vi "Test Comparison.vi"(8 "error in":errorcluster) -> (0 "error out":errorcluster)   [LabVIEW 2013]
uses:
  <vilib>/addons/_JKI Toolkits/Caraya/classes/Test/Test.lvclass
  <vilib>/addons/_JKI Toolkits/Caraya/classes/Assert/Assert.lvclass
  <vilib>/addons/_JKI Toolkits/Caraya/classes/Assert/Assert True.vi
  source/Timestamp Compare Units -- enum.ctl
  <vilib>/addons/_JKI Toolkits/Caraya/classes/Assert/Assert False.vi
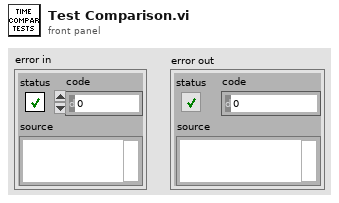
[diagram p1: front panel]
types:
  T1 = typedef "Timestamp Compare Units -- enum.ctl" = enum16{"week", "day", "hour", "minute", "second", "millisecond", "microsecond", "nanosecond"}
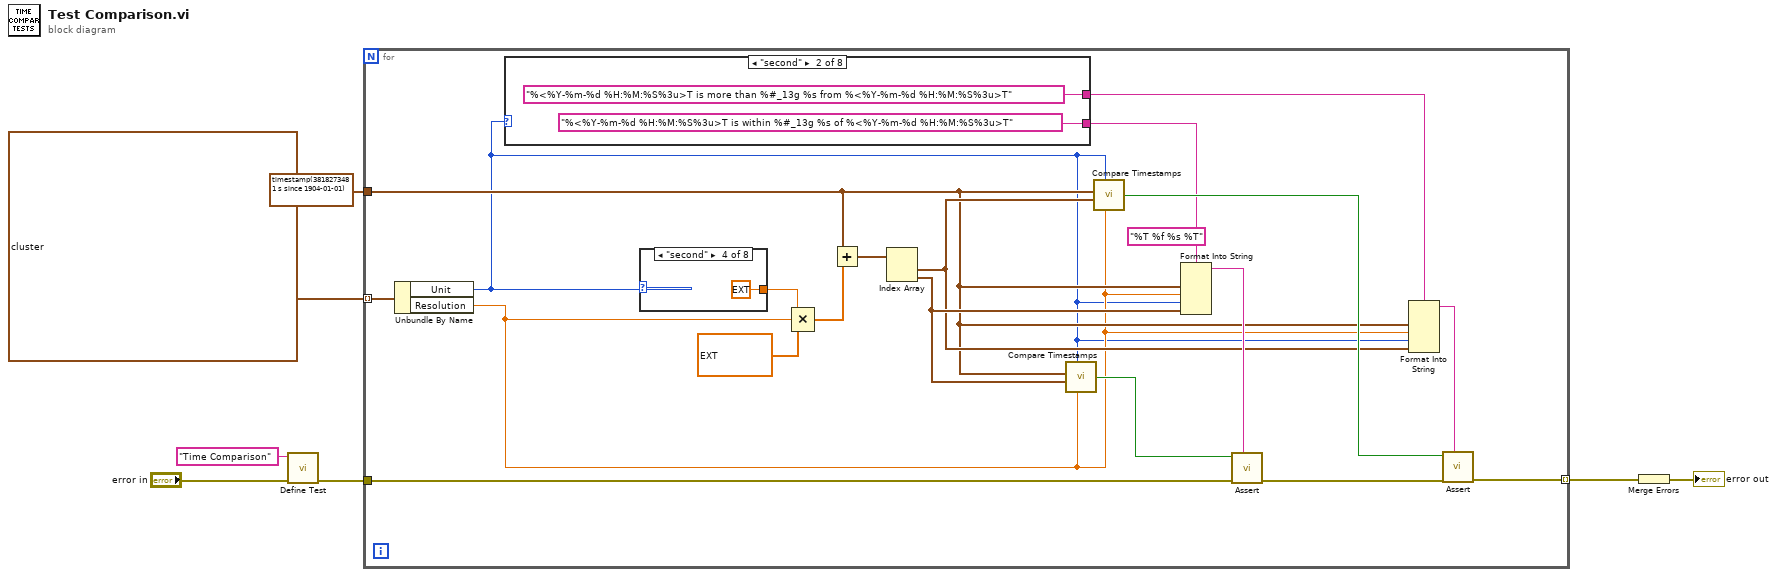
[diagram p0: block diagram]
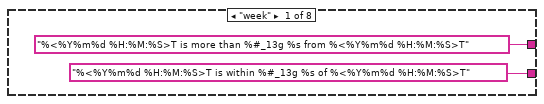
[diagram p2: hidden frame]
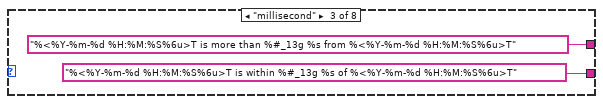
[diagram p3: hidden frame]
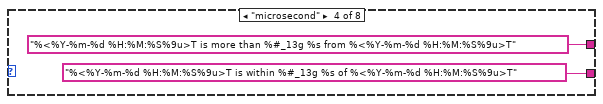
[diagram p4: hidden frame]
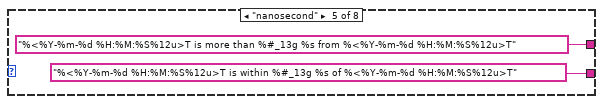
[diagram p5: hidden frame]
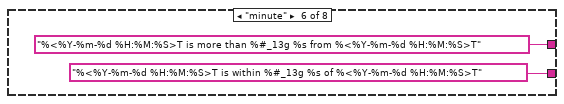
[diagram p6: hidden frame]
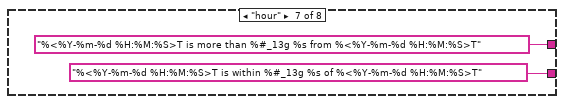
[diagram p7: hidden frame]
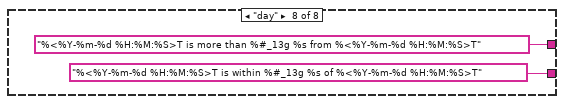
[diagram p8: hidden frame]
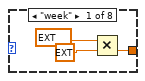
[diagram p9: hidden frame]
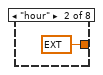
[diagram p10: hidden frame]
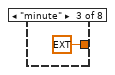
[diagram p11: hidden frame]
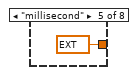
[diagram p12: hidden frame]
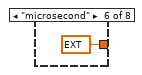
[diagram p13: hidden frame]
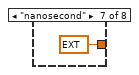
[diagram p14: hidden frame]
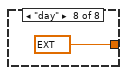
[diagram p15: hidden frame]
diagram:
  n1 = call <vilib>:"Define Test.vi"("error in (no error)"="error in", "Label (VI Title)"="Time Comparison") -> ("error out"=w2:errorcluster)  [unwired: 8 in, 1 out]
  n2 = for {
    tunnel: [w24] -> w4 mode=indexing
    tunnel: timestamp(3818273481.0647187 s since 1904-01-01) ("timestamp (1)") -> [w12]
    tunnel: w2 -> [w22]
    tunnel: cluster{"Resolution":ext, "Unit":T1}[] [{"Resolution"=1.0, "Unit"=enum."second"}, {"Resolution"=1.0, "Unit"=enum."millisecond"}, {"Resolution"=1.0, "Unit"=enum."microsecond"}, {"Resolution"=1.0, "Unit"=enum."minute"}, {"Resolution"=1.0, "Unit"=enum."day"}, {"Resolution"=0.05, "Unit"=enum."second"}] -> [w21] mode=indexing
    (unwired) "%T %f %s %T" ("format string")
    n3 = Unbundle By Name(w21) -> ("Unit"=w10:T1, "Resolution"=w11:ext)
    n4 = case shown="\"second\"" w10 {
      tunnel: ["%<%Y%m%d %H:%M:%S>T is within %#_13g %s of %<%Y%m%d %H:%M:%S>T" ("format string") "%<%Y-%m-%d %H:%M:%S%3u>T is within %#_13g %s of %<%Y-%m-%d %H:%M:%S%3u>T" ("format string") "%<%Y-%m-%d %H:%M:%S%6u>T is within %#_13g %s of %<%Y-%m-%d %H:%M:%S%6u>T" ("format string") "%<%Y-%m-%d %H:%M:%S%9u>T is within %#_13g %s of %<%Y-%m-%d %H:%M:%S%9u>T" ("format string") "%<%Y-%m-%d %H:%M:%S%12u>T is within %#_13g %s of %<%Y-%m-%d %H:%M:%S%12u>T" ("format string") "%<%Y-%m-%d %H:%M:%S>T is within %#_13g %s of %<%Y-%m-%d %H:%M:%S>T" ("format string") "%<%Y-%m-%d %H:%M:%S>T is within %#_13g %s of %<%Y-%m-%d %H:%M:%S>T" ("format string") "%<%Y-%m-%d %H:%M:%S>T is within %#_13g %s of %<%Y-%m-%d %H:%M:%S>T" ("format string")] -> w8
      tunnel: ["%<%Y%m%d %H:%M:%S>T is more than %#_13g %s from %<%Y%m%d %H:%M:%S>T" ("format string") "%<%Y-%m-%d %H:%M:%S%3u>T is more than %#_13g %s from %<%Y-%m-%d %H:%M:%S%3u>T" ("format string") "%<%Y-%m-%d %H:%M:%S%6u>T is more than %#_13g %s from %<%Y-%m-%d %H:%M:%S%6u>T" ("format string") "%<%Y-%m-%d %H:%M:%S%9u>T is more than %#_13g %s from %<%Y-%m-%d %H:%M:%S%9u>T" ("format string") "%<%Y-%m-%d %H:%M:%S%12u>T is more than %#_13g %s from %<%Y-%m-%d %H:%M:%S%12u>T" ("format string") "%<%Y-%m-%d %H:%M:%S>T is more than %#_13g %s from %<%Y-%m-%d %H:%M:%S>T" ("format string") "%<%Y-%m-%d %H:%M:%S>T is more than %#_13g %s from %<%Y-%m-%d %H:%M:%S>T" ("format string") "%<%Y-%m-%d %H:%M:%S>T is more than %#_13g %s from %<%Y-%m-%d %H:%M:%S>T" ("format string")] -> w9
      frame "week" {
      }
      frame "second" {
      }
      frame "millisecond" {
      }
      frame "microsecond" {
      }
      frame "nanosecond" {
      }
      frame "minute" {
      }
      frame "hour" {
      }
      frame "day" {
      }
    }
    n5 = case shown="\"second\"" w10 {
      tunnel: [w43 ext 3600.0 ("y") ext 60.0 ("y") ext 1.0 ("y") ext 0.00099999999999999999996 ("y") ext 0.00000100000000000000000004 ("y") ext 1e-9 ("y") ext 86400.0 ("y")] -> w20
      frame "week" {
        n6 = Multiply(x=ext 86400.0 ("y"), y=ext 4.0) -> (x*y=w43:ext)
      }
      frame "hour" {
      }
      frame "minute" {
      }
      frame "second" {
      }
      frame "millisecond" {
      }
      frame "microsecond" {
      }
      frame "nanosecond" {
      }
      frame "day" {
      }
    }
    n7 = Compound Arithmetic op=MULTIPLY(w20, w11, ext[] [1.1, 0.9]) -> (w18:ext[])
    n8 = Add(x=w12, y=w18) -> (x+y=w17:timestamp[])
    n9 = Index Array(array=w17) -> (element #1=w13:timestamp, element #2=w14:timestamp)  [unwired: 2 in]
    n10 = call "Compare Timestamps.vi"("Unit (ms)"=w10, "timestamp (1)"=w12, "timestamp (2)"=w14, "Resolution (in selected unit)"=w11) -> ("Equal?"=w26:bool)  [unwired: 4 in]
    n11 = call "Compare Timestamps.vi"("Unit (ms)"=w10, "timestamp (1)"=w12, "timestamp (2)"=w13, "Resolution (in selected unit)"=w11) -> ("Equal?"=w23:bool)  [unwired: 4 in]
    n12 = Format Into String(format string=w8, w12, w11, w10, w14) -> (resulting string=w16:string)  [unwired: 2 in, 1 out]
    n13 = call-poly <vilib>:"Assert.vi"("Label"=w16, "error in (no error)"=w22, "True?"=w26) -> ("error out"=w25:errorcluster)  [unwired: 7 in, 1 out]
    n14 = Format Into String(format string=w9, w12, w11, w10, w13) -> (resulting string=w15:string)  [unwired: 2 in, 1 out]
    n15 = call-poly <vilib>:"Assert.vi"("Label"=w15, "error in (no error)"=w25, "False?"=w23) -> ("error out"=w24:errorcluster)  [unwired: 7 in, 1 out]
  }
  n16 = Merge Errors(w4) -> (→"error out":errorcluster)
